vi "Control_ReadJoystick1.vi"() -> (4 "Up":bool, 6 "Down":bool, 8 "Left":bool, 10 "Right":bool, 15 "Button":bool)   [LabVIEW 2018]
uses:
  <vilib>/rvi/eio/common/nirviEmuTemplateMethod_errors.vi
  <vilib>/eio/EIONode/EIONode.xnode
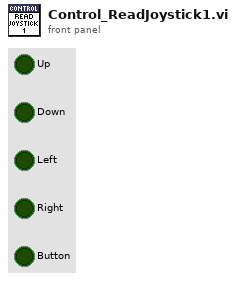
[diagram p1: front panel]
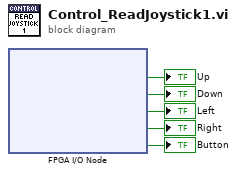
[diagram p0: block diagram]
diagram:
  n1 = xnode "FPGA I/O Node"() -> ("ConnectorA/DIO0"=→"Up":bool, "ConnectorA/DIO1"=→"Down":bool, "ConnectorA/DIO2"=→"Left":bool, "ConnectorA/DIO3"=→"Right":bool, "ConnectorA/DIO4"=→"Button":bool)  [unwired: 5 in, 5 out]
